vi "Helper Core.vi"(8 "error in (no error)":errorcluster, 10 "data":waveform(dbl)[](array[waveform]), 11 "Analog Reader Helper in":refnum<class "Analog Reader Helper.lvclass">) -> (0 "error out":errorcluster, 3 "Analog Reader Helper out":refnum<class "Analog Reader Helper.lvclass">)   [LabVIEW 2024, in "DAQmx Actor.lvlib" / "Analog Reader Helper.lvclass"]
uses:
  Analog Reader Helper.lvclass
  Analog Reader Helper.lvclass/Analog Reader Helper.ctl
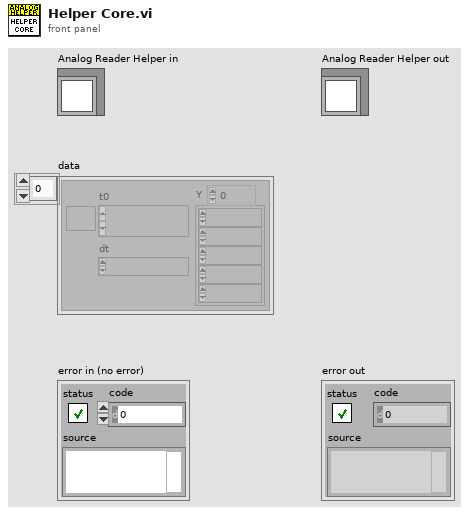
[diagram p1: front panel]
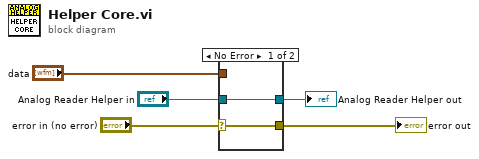
[diagram p0: block diagram]
diagram:
  n1 = case shown="No Error" "error in (no error)" {
    selector: "error in (no error)" -> [w6 w9]
    tunnel: [w6 w9] -> w4
    tunnel: [w7 w8] -> w2
    tunnel: "Analog Reader Helper in" -> [w7 w8]
    tunnel: "data" -> [_ _]
    frame No Error {
    }
    frame Error {
    }
  }
  "error out" <- w4
  "Analog Reader Helper out" <- w2
